vi "Tread_02.vi"(0 "IP":string="192.168.1.126", 1 "ID":u8=1, 2 "EnRefnum":refnum<vi>, 3 "StRefnum":refnum<vi>, 5 "Port":u16=1621, 9 "Number":u8=2, 11 "error in":errorcluster) -> (15 "error out":errorcluster)   [LabVIEW 2011]
uses:
  Enumerator/CmdType.ctl
  DLL/Certificate_02.vi
  Look-up/CardInfo/SPR_02.vi
  Look-up/Password/PSW_02.vi
  Queue/Door_02.vi
  Interface/SockeHook/Hook_02.vi
  Variable/gSTOP.vi
  DoorProc/DoorProc_02.vi
  Queue/Card.vi
  Interface/TimeOut/TimeOut_02.vi
  CmdParse/CmdParse_2.vi
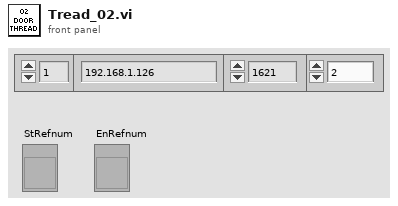
[diagram p1: front panel]
types:
  T1 = enum16{"Initial", "Insert", "Delete", "Search", "Release"}
  T2 = enum16{"Open", "Verify", "Password", "Log", "Close"}
  T3 = enum16{"Open", "R", "W", "R->W", "W->R", "Close"}
  T4 = enum16{"Obtain", "Enqueue", "Dequeue", "Release"}
  T5 = cluster{"Read Array":u8[], "Socket Id":u8, "Node Id":u8}
  T6 = typedef "CmdType.ctl" = enum16{"GetEventLog", "DelTransaction", "InvalidMessage", "RelayControl", "RelayOff", "RelayOn", "VaildMessage", "EventPolling", "StoppingWaiting", "PromptKeying-in"}
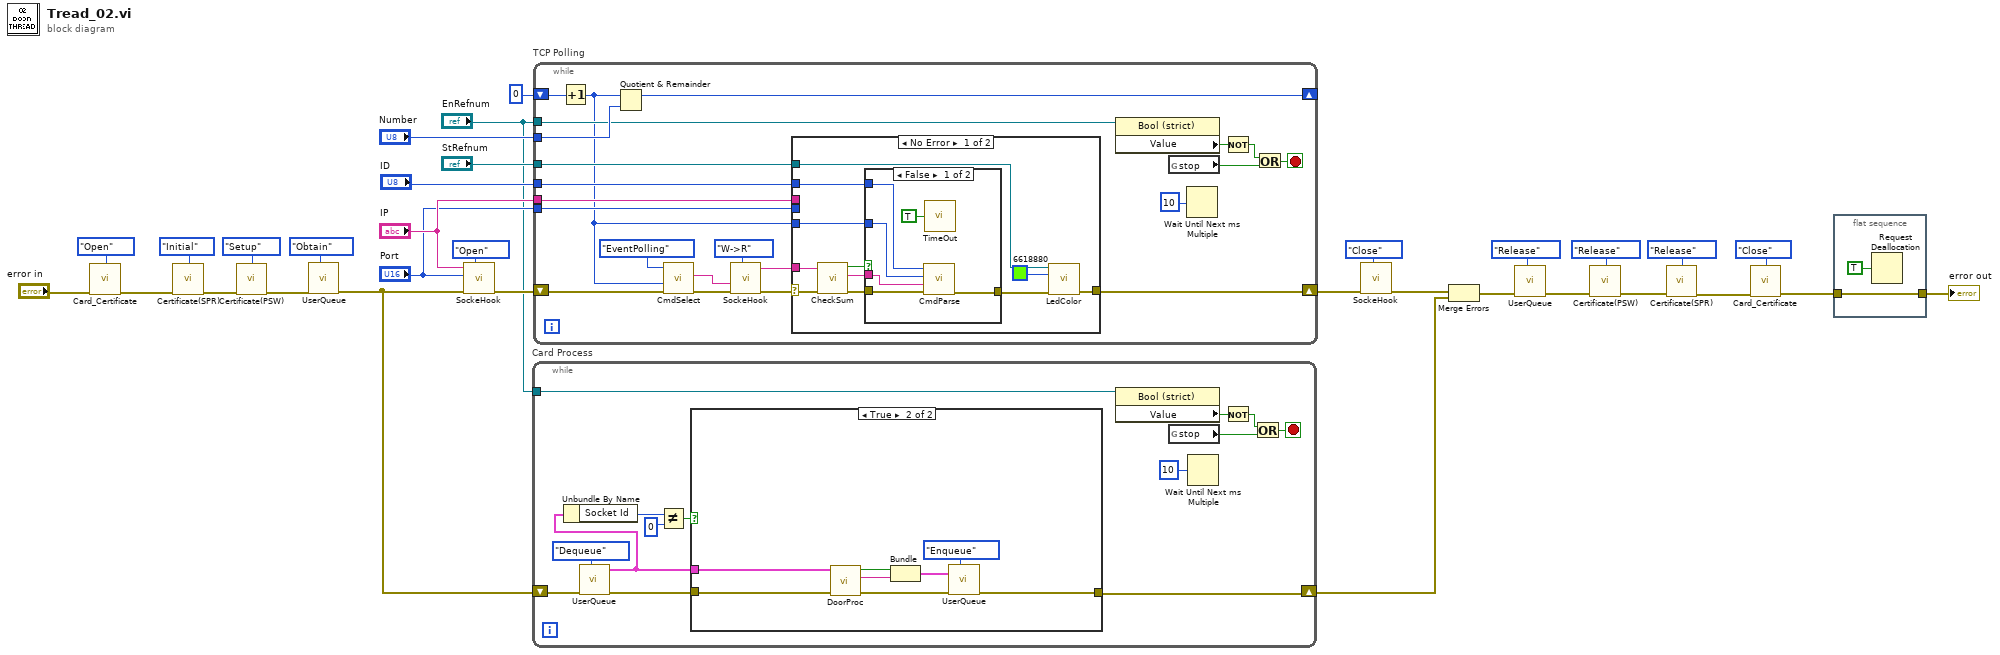
[diagram p0: block diagram]
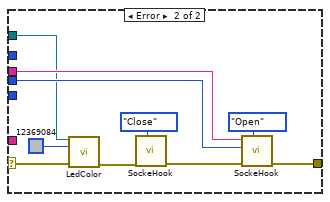
[diagram p3: hidden frame]
diagram:
  n1 = call-poly "Card_Certificate.vi"("DB"=T2."Open", "error in"="error in") -> ("error out"=w4:errorcluster)  [unwired: 12 in, 1 out]
  n2 = call-poly "Certificate(SPR).vi"("select"=T1."Initial", "error in"=w4) -> ("error out"=w10:errorcluster)  [unwired: 11 in, 2 out]
  n3 = call-poly "Certificate(PSW).vi"("select"=enum16{"Setup", "Search", "Release"}."Setup", "error in"=w10) -> ("error out"=w3:errorcluster)  [unwired: 11 in, 2 out]
  n4 = call-poly "UserQueue.vi"("Mode"=T4."Obtain", "error in (no error)"=w3) -> ("error out"=w27:errorcluster)  [unwired: 8 in, 1 out]
  n5 = call-poly "SockeHook.vi"("Mode"=T3."Open", "error in (no error)"=w27, "Port"="Port", "Machine"="IP") -> ("error out"=w22:errorcluster)  [unwired: 6 in, 1 out]
  n6 = while "Card Process" {
    shift-right: [w35] -> w32
    shift-left: w27 -> [w45]
    tunnel: "EnRefnum" -> [w37]
    stop <- w36 stop-if-true
    n7 = call-poly "UserQueue.vi"("Mode"=T4."Dequeue", "error in (no error)"=w45) -> ("error out"=w40:errorcluster, "Queue Out"=w39:T5)  [unwired: 8 in]
    n8 = Unbundle By Name(w39) -> ("Socket Id"=w44:u8)
    n9 = Not Equal?(x=w44, y=u8 0) -> (x != y?=w41:bool)
    n10 = case shown="True" w41 {
      tunnel: w40 -> [w47 w50]
      tunnel: [w47 w54] -> w35
      tunnel: w39 -> [_ w49]
      frame False {
      }
      frame True {
        n11 = call-poly "DoorProc.vi"("error in"=w50, "Cluster"=w49) -> ("error out"=w51:errorcluster, "Card Info"=w48:string, "Certificate"=w52:bool)  [unwired: 7 in]
        n12 = Bundle("Certificate"=w52, "Card Info"=w48) -> (w53:cluster{"Certificate":bool, "Card Info":string})  [unwired: 1 in]
        n13 = call-poly "UserQueue.vi"("Mode"=T4."Enqueue", "error in (no error)"=w51, "Queue In"=w53) -> ("error out"=w54:errorcluster)  [unwired: 7 in, 1 out]
      }
    }
    n14 = property class="Bool (strict)"(reference=w37) -> ("Value"=w38:bool)  [unwired: 1 in, 2 out]
    n15 = global read "gSTOP.vi" "stop"() -> (w33:bool)
    n16 = Wait Until Next ms Multiple(millisecond multiple=u32 10) -> ()  [unwired: 1 out]
    n17 = Not(x=w38) -> (.not. x?=w34:bool)
    n18 = Or(x=w34, y=w33) -> (x .or. y?=w36:bool)
  }
  n19 = while "TCP Polling" {
    tunnel: "IP" -> [w77]
    tunnel: "Port" -> [w76]
    tunnel: "ID" -> [w75]
    shift-right: [w59] -> w25
    shift-left: w22 -> [w74]
    shift-right: [w72] -> _
    shift-left: u8 0 -> [w71]
    tunnel: "Number" -> [w64]
    tunnel: "StRefnum" -> [w63]
    tunnel: "EnRefnum" -> [w62]
    stop <- w60 stop-if-true
    n20 = Increment(x=w71) -> (x+1=w56:u8)
    n21 = Quotient & Remainder(x=w56, y=w64) -> (x-y*floor(x/y)=w72:u8)  [unwired: 1 out]
    n22 = call "CmdSelect.vi"("error in (no error)"=w74, "Node Id"=w56, "Cmd Type"=CmdType."EventPolling" ("cmd type in")) -> ("error out"=w69:errorcluster, "Cmd Str"=w68:string)  [unwired: 7 in]
    n23 = call-poly "SockeHook.vi"("Mode"=T3."W->R", "error in (no error)"=w69, "data in"=w68) -> ("error out"=w66:errorcluster, "data out"=w67:string)  [unwired: 7 in]
    n24 = case shown="No Error" w66 {
      selector: w66 -> [w86 w99]
      tunnel: [w80 w104] -> w59
      tunnel: w77 -> [_ w103]
      tunnel: w76 -> [_ w102]
      tunnel: w67 -> [w83 _]
      tunnel: w75 -> [w87 _]
      tunnel: w63 -> [w79 w97]
      tunnel: w56 -> [w78 _]
      frame No Error {
        n25 = call "CheckSum.vi"("error in (no error)"=w86, "string in"=w83) -> ("error out"=w85:errorcluster, "string out"=w84:string, "No Parse"=w88:bool)  [unwired: 7 in]
        n26 = case shown="False" w88 {
          tunnel: w87 -> [w94 _]
          tunnel: w85 -> [w93 w95]
          tunnel: [w92 w95] -> w81
          tunnel: w84 -> [w91 _]
          tunnel: w78 -> [w89 _]
          frame False {
            n27 = call-poly "CmdParse.vi"("error in (no error)"=w93, "Read Buffer"=w91, "Node Id"=w89, "Socket Id"=w94) -> ("error out"=w92:errorcluster)  [unwired: 7 in]
            n28 = call-poly "TimeOut.vi"("Reset"=TRUE) -> ()  [unwired: 4 in, 1 out]
          }
          frame True {
          }
        }
        n29 = call "LedColor.vi"("Boolean in"=w79, "Color Box"=u32 6618880, "error in (no error)"=w81) -> ("error out"=w80:errorcluster)  [unwired: 12 in]
      }
      frame Error {
        n30 = call "LedColor.vi"("Boolean in"=w97, "Color Box"=u32 12369084, "error in (no error)"=w99) -> ("error out"=w98:errorcluster)  [unwired: 12 in]
        n31 = call-poly "SockeHook.vi"("Mode"=T3."Close", "error in (no error)"=w98) -> ("error out"=w105:errorcluster)  [unwired: 8 in, 1 out]
        n32 = call-poly "SockeHook.vi"("Mode"=T3."Open", "error in (no error)"=w105, "Port"=w102, "Machine"=w103) -> ("error out"=w104:errorcluster)  [unwired: 6 in, 1 out]
      }
    }
    n33 = property class="Bool (strict)"(reference=w62) -> ("Value"=w61:bool)  [unwired: 1 in, 2 out]
    n34 = global read "gSTOP.vi" "stop"() -> (w57:bool)
    n35 = Wait Until Next ms Multiple(millisecond multiple=u32 10) -> ()  [unwired: 1 out]
    n36 = Not(x=w61) -> (.not. x?=w58:bool)
    n37 = Or(x=w58, y=w57) -> (x .or. y?=w60:bool)
  }
  n38 = call-poly "SockeHook.vi"("Mode"=T3."Close", "error in (no error)"=w25) -> ("error out"=w31:errorcluster)  [unwired: 8 in, 1 out]
  n39 = Merge Errors(w31, w32) -> (w30:errorcluster)
  n40 = call-poly "UserQueue.vi"("Mode"=T4."Release", "error in (no error)"=w30) -> ("error out"=w2:errorcluster)  [unwired: 8 in, 1 out]
  n41 = call-poly "Certificate(PSW).vi"("select"=enum16{"Setup", "Search", "Release"}."Release", "error in"=w2) -> ("error out"=w7:errorcluster)  [unwired: 11 in, 2 out]
  n42 = call-poly "Certificate(SPR).vi"("select"=T1."Release", "error in"=w7) -> ("error out"=w1:errorcluster)  [unwired: 11 in, 2 out]
  n43 = call-poly "Card_Certificate.vi"("DB"=T2."Close", "error in"=w1) -> ("error out"=w14:errorcluster)  [unwired: 12 in, 1 out]
  n44 = flat-sequence {
    tunnel: w14 -> [w106]
    tunnel: [w106] -> w13
    frame #0 {
      n45 = Request Deallocation(TRUE ("flag")) -> ()
    }
  }
  "error out" <- w13
